vi "VSMMagnetMonitor.vi"() -> ()   [LabVIEW 2019]
uses:
  Utility/VSM/VSM9T-Cluster.ctl
  Instrument_Setup.vi
  Global/Global Variables/Data_Display_global.vi
panel:
  in  "stop":bool
  out "VSM-9T-Cluster":T1 {"Rate (T/min)" format="%6_5f"; "Leads (T)" format="%6_5f"}
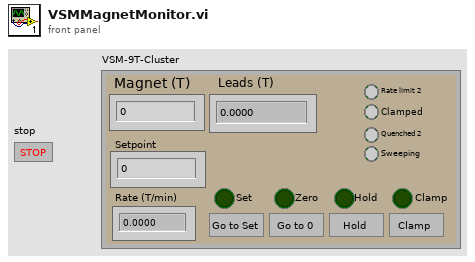
[diagram p1: front panel]
types:
  T1 = typedef "VSM9T-Cluster.ctl" = cluster{"Go to set":bool, "Go to Zero":bool, "Clamp":bool, "Go to Hold":bool, "Clamped ":bool, "Quenched 2":bool, "Rate limit 2":bool, "Magnet (T)":dbl, "Leads (T)":dbl, "Rate (T/min)":dbl, "Sweeping":bool, "Setpoint":dbl, "Set":bool, "Zero":bool, "Hold":bool, "Clamp":bool}
  T2 = typedef "PSIO.ctl" = cluster{"Address":T3, "Version":enum16{"PS", "IPS"}}
  T3 = typedef "OxfordAddress.ctl" = cluster{"Com Port":i32, "ISOBUS Address":i32, "GPIB Address":i16, "Communication":enum16{"RS232", "ISOBUS", "GPIB", "Gateway"}}
  T4 = cluster{"Version\n":string, "Max Sweep":dbl[unit], "Max Field":dbl[unit], "IO Info":T2}
  T5 = cluster{"Value":i16, "At rest":bool, "Sweeping":bool, "Rate limiting":bool}
  T6 = cluster{"Value":i16, "Hold":bool, "To set point":bool, "To zero":bool, "Clamped":bool}
  T7 = cluster{"Value":i16, "Desired":u16, "Magnet":u16, "Commanded":u16, "Actual":u16}
  T8 = cluster{"Value":i16, "Quenched":bool, "Over heated":bool, "Warming up":bool}
  T9 = typedef "VSM9T-Control-Cluster.ctl" = cluster{"Go to set":bool, "Go to Zero":bool, "Clamp":bool, "Go to Hold":bool, "Rate (T/min)":dbl, "Setpoint":dbl}
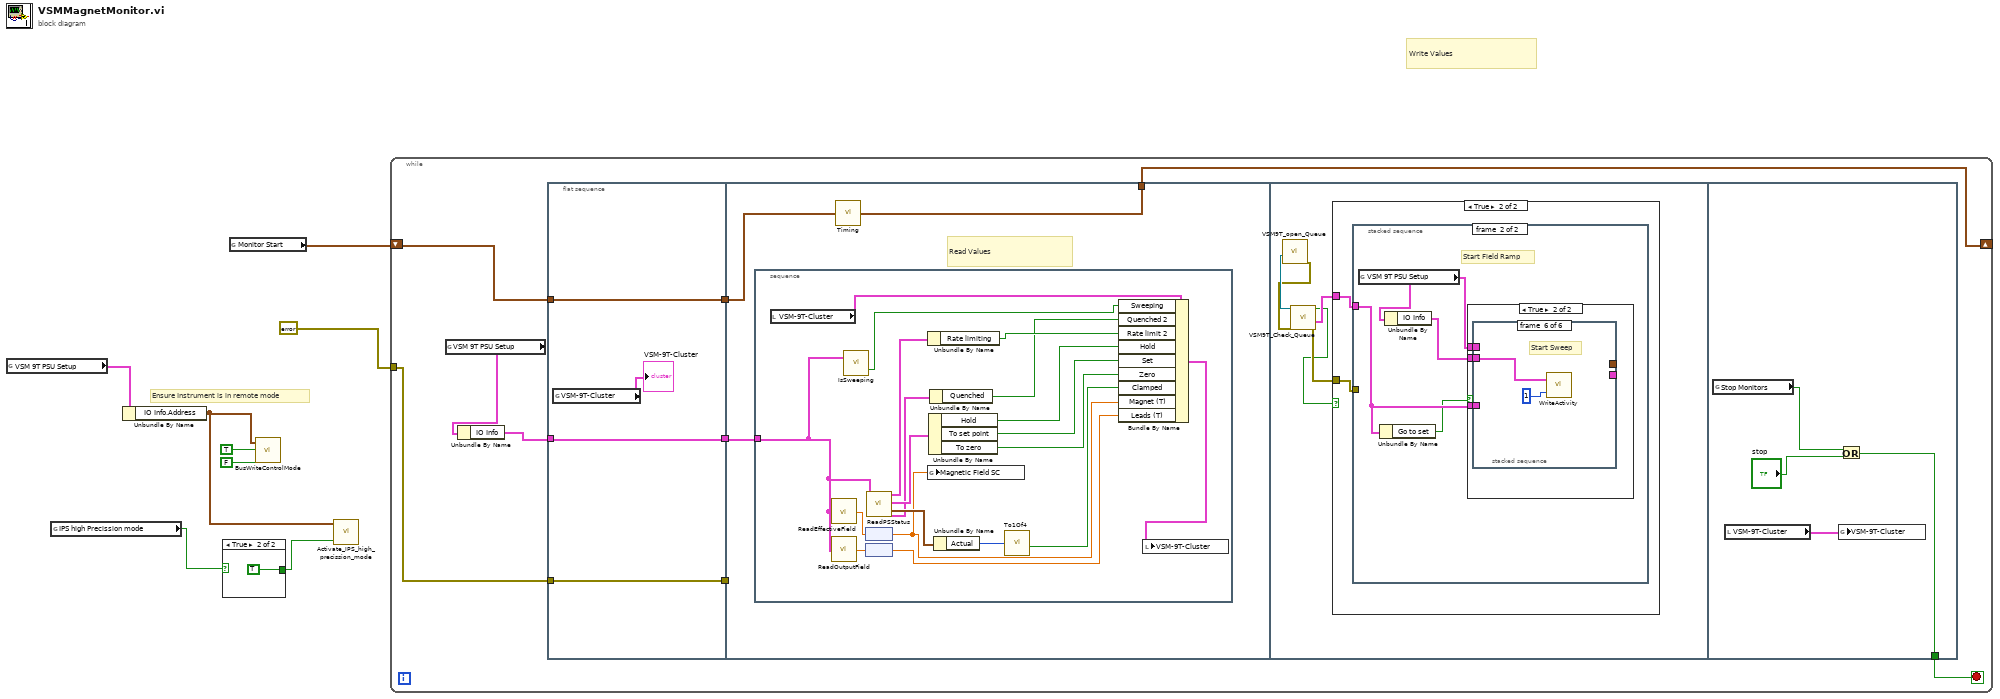
[diagram p0: block diagram]
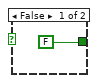
[diagram p2: hidden frame]
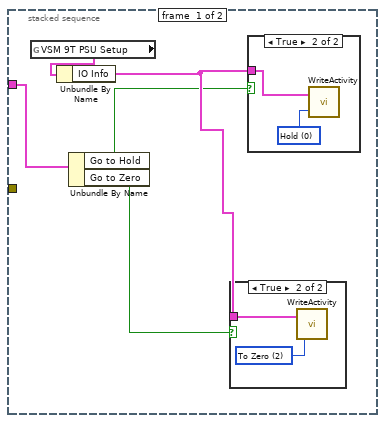
[diagram p4: hidden frame]
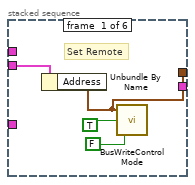
[diagram p8: hidden frame]
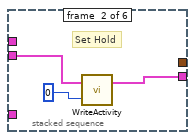
[diagram p9: hidden frame]
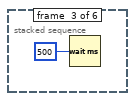
[diagram p10: hidden frame]
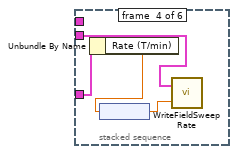
[diagram p11: hidden frame]
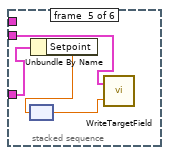
[diagram p12: hidden frame]
diagram:
  # "Ensure Instrument is in remote mode"
  # "Write Values"
  n1 = global read "Instrument_Setup.vi" "VSM 9T PSU Setup"() -> (w7:T4)
  n2 = global read "Instrument_Setup.vi" "IPS high Precission mode"() -> (w2:bool)
  n3 = Unbundle By Name(w7) -> ("IO Info.Address"=w1:T3)
  n4 = case shown="True" w2 {
    tunnel: [FALSE TRUE] -> w3
    frame False {
    }
    frame True {
    }
  }
  n5 = global read "Data_Display_global.vi" "Monitor Start"() -> (w4:timestamp)
  n6 = call "BusWriteControlMode.vi"("Locked"=FALSE, "Remote"=TRUE, "Address"=w1) -> ()  [unwired: 1 out]
  n7 = call "Activate_IPS_high_precission_mode.vi"("High Precission"=w3, "Address"=w1) -> ()  [unwired: 1 in, 1 out]
  n8 = while {
    tunnel: errorcluster {"status"=FALSE, "code"=0, "source"=""} ("error constant") -> [w19]
    shift-right: [w17] -> _
    shift-left: w4 -> [w18]
    stop <- w16 stop-if-true
    n9 = global read "Instrument_Setup.vi" "VSM 9T PSU Setup"() -> (w14:T4)
    n10 = Unbundle By Name(w14) -> ("IO Info"=w15:T2)
    n11 = flat-sequence {
      tunnel: w15 -> [w21]
      tunnel: w18 -> [w22]
      tunnel: w19 -> [w23]
      tunnel: [w23] -> w13
      tunnel: [w22] -> w12
      tunnel: [w21] -> w11
      tunnel: [w26] -> w17
      tunnel: w13 -> [_]
      tunnel: w12 -> [w25]
      tunnel: w11 -> [w24]
      tunnel: [w87] -> w16
      frame #0 {
        n12 = global read "Data_Display_global.vi" "VSM-9T-Cluster"() -> (→"VSM-9T-Cluster":T1)
      }
      frame #1 {
        # "Read Values"
        n13 = stacked-sequence {
          tunnel: w24 -> [w39]
          frame #0 {
            n14 = local read "VSM-9T-Cluster"() -> (w37:T1)
            n15 = call "ReadEffectiveField.vi"("IO Info"=w39) -> ("Effective field"=w40:dbl[unit])  [unwired: 2 out]
            n16 = call "ReadOutputField.vi"("IO Info"=w39) -> ("Field"=w41:dbl[unit])  [unwired: 2 out]
            n17 = call "IsSweeping.vi"("IO Info"=w39) -> ("Sweeping"=w34:bool)  [unwired: 1 in, 1 out]
            n18 = node(w40) -> (w28:dbl)
            n19 = node(w41) -> (w27:dbl)
            n20 = call "ReadPSStatus.vi"("IO Info"=w39) -> ("Mode (n)"=w44:T5, "Activity"=w45:T6, "Polarity"=w43:T7, "System Status (m)"=w42:T8)  [unwired: 10 in, 5 out]
            n21 = Unbundle By Name(w44) -> ("Rate limiting"=w35:bool)
            n22 = global write "Data_Display_global.vi" "Magnetic Field SC"(w28) -> ()
            n23 = Unbundle By Name(w45) -> ("Hold"=w32:bool, "To set point"=w31:bool, "To zero"=w30:bool)
            n24 = Unbundle By Name(w42) -> ("Quenched"=w33:bool)
            n25 = Unbundle By Name(w43) -> ("Actual"=w38:u16)
            n26 = call "To1Of4.vi"("Input"=w38) -> ("3"=w29:bool)  [unwired: 3 out]
            n27 = Bundle By Name(cluster=w37, "Sweeping"=w34, "Quenched 2"=w33, "Rate limit 2"=w35, "Hold"=w32, "Set"=w31, "Zero"=w30, "Clamped"=w29, "Magnet (T)"=w28, "Leads (T)"=w27) -> (w36:T1)
            n28 = local write "VSM-9T-Cluster"(w36) -> ()
          }
        }
        n29 = call "Timing.vi"("start time (s)"=w25) -> ("last reading (s)"=w26:timestamp)
      }
      frame #2 {
        n30 = call "VSM9T_open_Queue.vi"() -> ("error out"=w49:errorcluster, "queue out"=w50:refnum<queue>)  [unwired: 10 in]
        n31 = call "VSM9T_Check_Queue.vi"("error in (no error)"=w49, "Queue"=w50) -> ("error out"=w48:errorcluster, "VSM-9T-Control-Cluster"=w47:T9, "New Entries?"=w46:bool)  [unwired: 6 in]
        n32 = case shown="True" w46 {
          tunnel: w48 -> [_ w52]
          tunnel: w47 -> [_ w51]
          frame False {
          }
          frame True {
            n33 = stacked-sequence {
              tunnel: w52 -> [_ _]
              tunnel: w51 -> [w55 w63]
              frame #0 {
                n34 = global read "Instrument_Setup.vi" "VSM 9T PSU Setup"() -> (w57:T4)
                n35 = Unbundle By Name(w57) -> ("IO Info"=w56:T2)
                n36 = Unbundle By Name(w55) -> ("Go to Hold"=w54:bool, "Go to Zero"=w53:bool)
                n37 = case shown="True" w53 {
                  tunnel: w56 -> [_ w59]
                  frame False {
                  }
                  frame True {
                    w58 = u16 2 items=["Hold", "To Set Point", "To Zero", "Clamp"] ("Activity")
                    n38 = call "WriteActivity.vi"("Activity"=w58, "IO Info"=w59) -> ()  [unwired: 1 in, 1 out]
                  }
                }
                n39 = case shown="True" w54 {
                  tunnel: w56 -> [_ w61]
                  frame False {
                  }
                  frame True {
                    w60 = u16 0 items=["Hold", "To Set Point", "To Zero", "Clamp"] ("Activity")
                    n40 = call "WriteActivity.vi"("Activity"=w60, "IO Info"=w61) -> ()  [unwired: 1 in, 1 out]
                  }
                }
              }
              frame #1 {
                # "Start Field Ramp"
                n41 = global read "Instrument_Setup.vi" "VSM 9T PSU Setup"() -> (w64:T4)
                n42 = Unbundle By Name(w63) -> ("Go to set"=w62:bool)
                n43 = Unbundle By Name(w64) -> ("IO Info"=w65:T2)
                n44 = case shown="True" w62 {
                  tunnel: w65 -> [_ w68]
                  tunnel: w64 -> [_ w67]
                  tunnel: w63 -> [_ w66]
                  frame False {
                  }
                  frame True {
                    n45 = stacked-sequence {
                      tunnel: [_ w75 _ _ _ _] -> _
                      tunnel: w68 -> [w70 w73 _ w79 w81 w85]
                      tunnel: [w69 _ _ _ _ _] -> _
                      tunnel: w67 -> [_ _ _ _ _ _]
                      tunnel: w66 -> [_ _ _ w80 w84 _]
                      frame #0 {
                        # "Set Remote"
                        n46 = Unbundle By Name(w70) -> ("Address"=w69:T3)
                        n47 = call "BusWriteControlMode.vi"("Locked"=FALSE, "Remote"=TRUE, "Address"=w69) -> ()  [unwired: 1 out]
                      }
                      frame #1 {
                        # "Set Hold"
                        n48 = call "WriteActivity.vi"("Activity"=0, "IO Info"=w73) -> ("IO Info"=w75:T2)  [unwired: 1 in]
                      }
                      frame #2 {
                        n49 = Wait (ms)(milliseconds to wait=u32 500) -> ()  [unwired: 1 out]
                      }
                      frame #3 {
                        n50 = Unbundle By Name(w80) -> ("Rate (T/min)"=w78:dbl)
                        n51 = node(w78) -> (w77:dbl[unit])
                        n52 = call "WriteFieldSweepRate.vi"("Sweep rate"=w77, "IO Info"=w79) -> ()  [unwired: 1 out]
                      }
                      frame #4 {
                        n53 = Unbundle By Name(w84) -> ("Setpoint"=w83:dbl)
                        n54 = node(w83) -> (w82:dbl[unit])
                        n55 = call "WriteTargetField.vi"("Target Field"=w82, "IO Info"=w81) -> ()  [unwired: 1 in, 1 out]
                      }
                      frame #5 {
                        # "Start Sweep"
                        n56 = call "WriteActivity.vi"("Activity"=1, "IO Info"=w85) -> ()  [unwired: 1 in, 1 out]
                      }
                    }
                  }
                }
              }
            }
          }
        }
      }
      frame #3 {
        n57 = global read "Data_Display_global.vi" "Stop Monitors"() -> (w89:bool)
        n58 = local read "VSM-9T-Cluster"() -> (w90:T1)
        n59 = global write "Data_Display_global.vi" "VSM-9T-Cluster"(w90) -> ()
        n60 = Or(x=w89, y="stop") -> (x .or. y?=w87:bool)
      }
    }
  }
